vi "FT10_FPGA_7854R Ask Dialog - Set Config.vi"(11 "7854 Set Config":T1) -> (3 "Set Config Out":bool)   [LabVIEW 2024]
uses:
  Controls/Control_PXI-7854R Set Config Bool.ctl
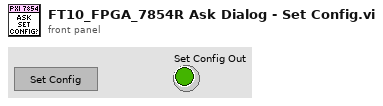
[diagram p1: front panel]
types:
  T1 = typedef "Control_PXI-7854R Set Config Bool.ctl" = bool
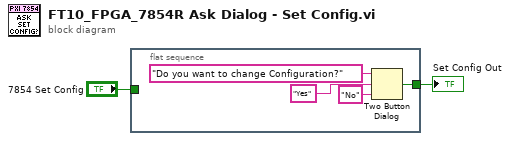
[diagram p0: block diagram]
diagram:
  n1 = flat-sequence {
    tunnel: [w3] -> w2
    tunnel: "7854 Set Config" -> [_]
    frame #0 {
      n2 = Two Button Dialog(message="Do you want to change Configuration?", 1:"No" ("F button name (\"Cancel\")"), 2:"Yes" ("T button name (\"OK\")")) -> (T button?=w3:bool)
    }
  }
  "Set Config Out" <- w2
